vi "NI VeriStand - Open Engine State Change Notification.vi"(8 "error in (no error)":errorcluster, 11 "WorkspaceManager in":T3) -> (0 "error out":errorcluster, 1 "SystemStateRefs":T2, 2 "SystemChangeEventRef":T1, 3 "WorkspaceManager out":T3)   [LabVIEW 2020, in "NI_VS Workspace ExecutionAPI.lvlib"]
doc: "Creates a reference to a user event that you can use to monitor the state of the VeriStand Engine."
uses:
  <vilib>/NI VeriStand/Execution/Workspace/NI_VS Workspace ExecutionAPI.lvlib
  <vilib>/NI VeriStand/Execution/Workspace/WorkspaceAPI.ctl
  NationalInstruments.VeriStand.ClientAPI
  <vilib>/NI VeriStand/Execution/Workspace/SystemStateEventRef.ctl
  <vilib>/NI VeriStand/Execution/Workspace/Target State Info.ctl
  <vilib>/NI VeriStand/Execution/Workspace/Target State.ctl
  <vilib>/NI VeriStand/Execution/Workspace/SystemStateRegEventRef.ctl
  <vilib>/NI VeriStand/Execution/Workspace/Target State Change Event Callback.vi
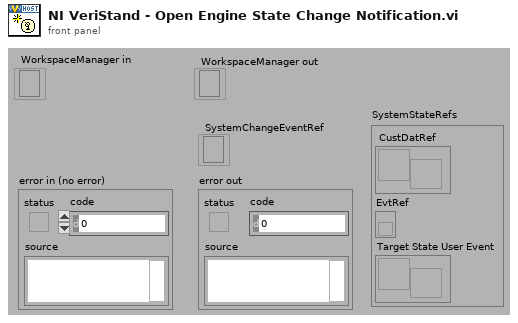
[diagram p1: front panel]
types:
  T1 = typedef "NI_VS Workspace ExecutionAPI.lvlib/SystemStateRegEventRef.ctl" = refnum<event-registration>
  T2 = typedef "NI_VS Workspace ExecutionAPI.lvlib/SystemStateEventRef.ctl" = cluster{"CustDatRef":refnum<user-event>, "EvtRef":refnum<k27>, "Target State User Event":refnum<user-event>}
  T3 = typedef "NI_VS Workspace ExecutionAPI.lvlib/WorkspaceAPI.ctl" = refnum<k24>
  T4 = typedef "NI_VS Workspace ExecutionAPI.lvlib/Target State Info.ctl" = cluster{"Target":string, "State":T5}
  T5 = typedef "NI_VS Workspace ExecutionAPI.lvlib/Target State.ctl" = enum16{"Disconnected", "Running", "Idle", "Disabled", "Connecting"}
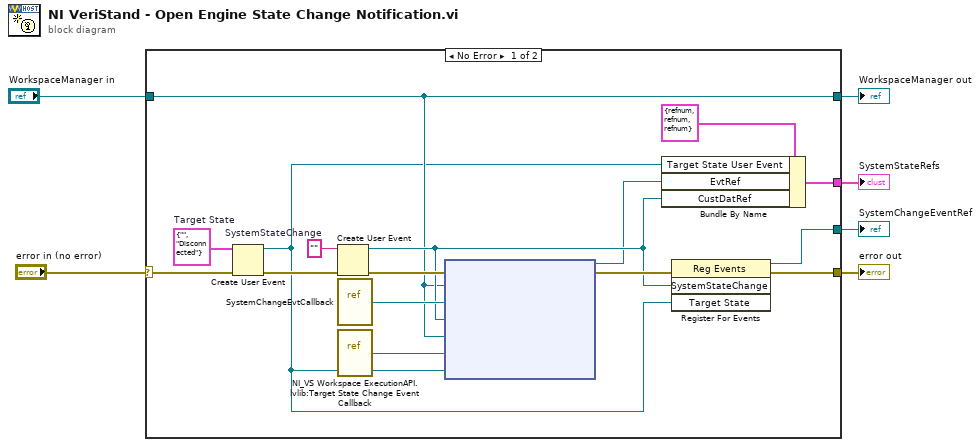
[diagram p0: block diagram]
diagram:
  n1 = case shown="No Error" "error in (no error)" {
    selector: "error in (no error)" -> [w12 w24]
    tunnel: [w19 _] -> w6
    tunnel: "WorkspaceManager in" -> [w9 w23]
    tunnel: [w11 w24] -> w3
    tunnel: [w10 _] -> w2
    tunnel: [w9 w23] -> w1
    frame No Error {
      w13 = T4 {"Target"="", "State"=enum."Disconnected"}  # Target State
      w20 = ""  # SystemStateChange
      n2 = Create User Event(user event datatype=w13, error in=w12) -> (user event=w8:refnum<user-event>, error out=w21:errorcluster)
      n3 = Create User Event(user event datatype=w20, error in=w21) -> (user event=w15:refnum<user-event>, error out=w17:errorcluster)
      n4 = vi-ref <vilib>:"SystemChangeEvtCallback.vi"() -> (w16:refnum<vi>)
      n5 = vi-ref "NI_VS Workspace ExecutionAPI.lvlib:Target State Change Event Callback.vi"() -> (w14:refnum<vi>)
      n6 = node(w17, w9, w16, w15, w9, w14, w8) -> (w7:refnum<k27>, w22:errorcluster)  [unwired: 1 in]
      n7 = Bundle By Name(cluster=T2 {"CustDatRef"=refnum, "EvtRef"=refnum, "Target State User Event"=refnum} ("SystemChangeRefs"), "Target State User Event"=w8, "EvtRef"=w7, "CustDatRef"=w15) -> (w19:T2)
      n8 = register-events(error in=w22, w15, w8) -> (reference out=w10:refnum<event-registration>, error out=w11:errorcluster)  [unwired: 1 in]
    }
    frame Error {
    }
  }
  "WorkspaceManager out" <- w1
  "error out" <- w3
  "SystemStateRefs" <- w6
  "SystemChangeEventRef" <- w2
